vi "FPGA_I2C_Write Byte.vi"(8 "Data":u8, 9 "Wait Time/2":u32, 10 "Wait Time":u32, 11 "IO Cluster":T1) -> (2 "Done?":bool, 3 "Ack":bool)   [LabVIEW 2020]
doc: "Writes a single byte to an I2C slave device on a single port."
uses:
  Controls/FPGA_I2C IO Cluster.ctl
  Controls/FPGA I2C_Write Byte State.ctl
  <vilib>/rvi/eio/common/nirviEmuTemplateMethod_errors.vi
  <vilib>/eio/EIOMethodNode/EIOMethodNode.xnode
  <vilib>/eio/EIONode/EIONode.xnode
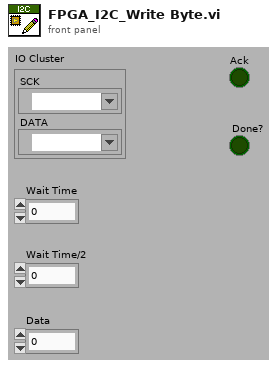
[diagram p1: front panel]
types:
  T1 = typedef "FPGA_I2C IO Cluster.ctl" = cluster{"SCK":refnum<k21>, "DATA":refnum<k21>}
  T2 = typedef "FPGA I2C_Write Byte State.ctl" = enum16{"Latch DATA", "Set DATA", "Wait Half 1", "Set SCK High 1", "Wait 1", "Set SCK Low 1", "Wait Half 2", "Release DATA", "Wait Half 3", "Set SCK High 2", "Wait Half 4", "Read Ack Bit", "Wait Half 5", "Set SCK Low 2", "Wait 2", "Stop"}
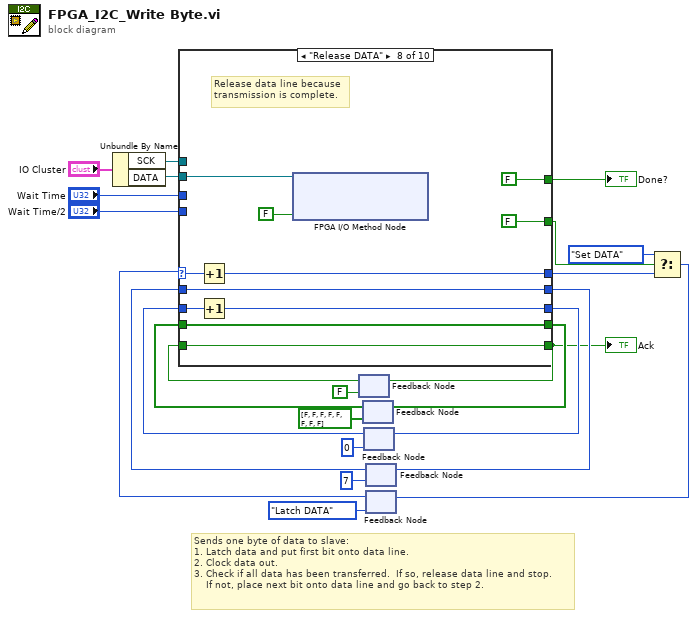
[diagram p0: block diagram]
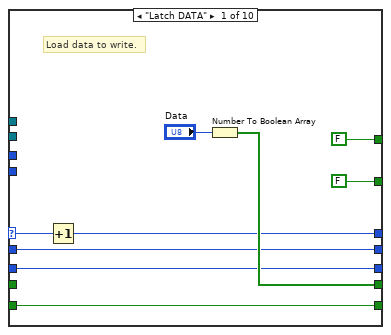
[diagram p2: hidden frame]
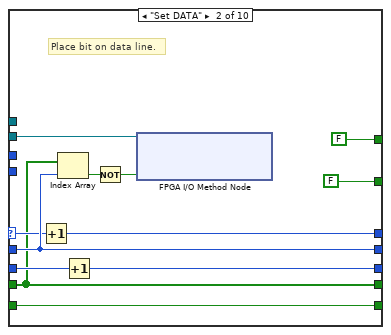
[diagram p3: hidden frame]
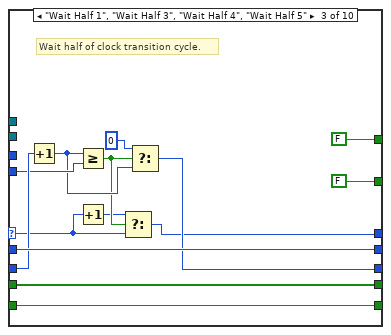
[diagram p4: hidden frame]
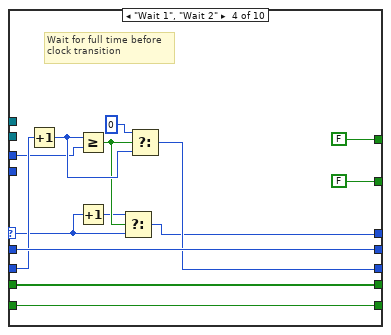
[diagram p5: hidden frame]
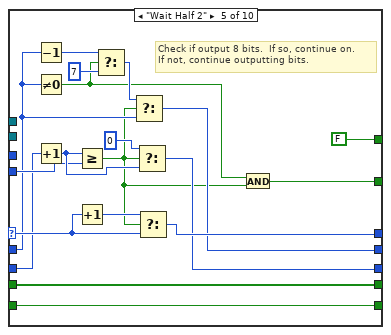
[diagram p6: hidden frame]
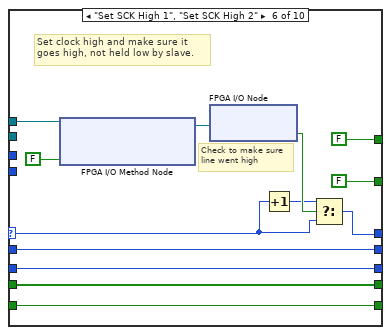
[diagram p7: hidden frame]
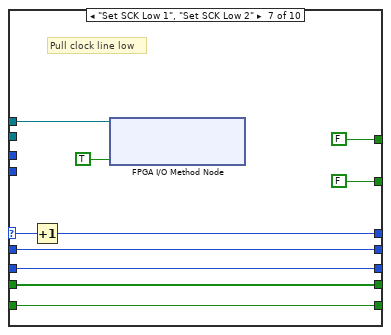
[diagram p8: hidden frame]
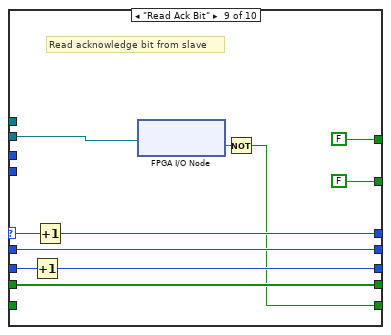
[diagram p9: hidden frame]
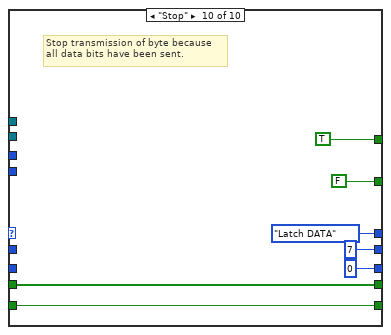
[diagram p10: hidden frame]
diagram:
  # "Sends one byte of data to slave:\n1. Latch data and put first bit onto data line.\n2. Clock data out.\n3. Check if all data has been transferred.  If so, release data line and stop.\n    If not, place next bit onto data line and go back to step 2."
  n1 = Unbundle By Name("IO Cluster") -> ("SCK"=w9:refnum<k21>, "DATA"=w10:refnum<k21>)
  n2 = feedback #1(FALSE) -> (w2:bool)
  n3 = feedback #2(bool[] [FALSE, FALSE, FALSE, FALSE, FALSE, FALSE, FALSE, FALSE] ("Boolean array")) -> (w6:bool[])
  n4 = feedback #3(u32 0) -> (w16:u32)
  n5 = feedback #4(i16 7) -> (w23:i16)
  n6 = feedback #5(FPGA_I2C_Write_Byte_State."Latch DATA" ("Enum")) -> (w4:T2)
  n7 = case shown="\"Release DATA\"" w4 {
    selector: w4 -> [w31 w42 w51 w66 w87 w103 w114 w123 w136 _]
    tunnel: w23 -> [w29 w44 w59 w73 w81 w105 w115 w126 w137 _]
    tunnel: [w29 w44 w59 w73 w80 w105 w115 w126 w137 i16 7 ("f")] -> w22
    tunnel: [FALSE FALSE FALSE FALSE w77 FALSE FALSE FALSE FALSE FALSE] -> w18
    tunnel: [FALSE FALSE FALSE FALSE FALSE FALSE FALSE FALSE FALSE TRUE] -> w20
    tunnel: [w28 w39 w54 w69 w83 w100 w111 w124 w133 u32 0 ("t")] -> w17
    tunnel: w16 -> [w28 w43 w58 w72 w84 w100 w111 w125 w134 _]
    tunnel: "Wait Time/2" -> [_ _ w57 _ w85 _ _ _ _ _]
    tunnel: [w30 w41 w50 w65 w86 w101 w113 w122 w135 FPGA_I2C_Write_Byte_State."Latch DATA" ("Enum")] -> w14
    tunnel: "Wait Time" -> [_ _ _ w64 _ _ _ _ _ _]
    tunnel: w10 -> [_ w38 _ _ _ _ _ w120 w132 _]
    tunnel: w9 -> [_ _ _ _ _ w95 w110 _ _ _]
    tunnel: [w32 w37 w49 w63 w76 w99 w109 w119 w131 w140] -> w7
    tunnel: w6 -> [_ w37 w49 w63 w76 w99 w109 w119 w131 w140]
    tunnel: w2 -> [w25 w34 w46 w60 w74 w93 w106 w116 _ w138]
    tunnel: [w25 w34 w46 w60 w74 w93 w106 w116 w127 w138] -> w1
    frame "Latch DATA" {
      # "Load data to write."
      n8 = Increment(x=w31) -> (x+1=w30:T2)
      n9 = Number To Boolean Array(number="Data") -> (Boolean array=w32:bool[])
    }
    frame "Set DATA" {
      # "Place bit on data line."
      n10 = Increment(x=w42) -> (x+1=w41:T2)
      n11 = Index Array(array=w37, index=w44) -> (element=w45:bool)
      n12 = Increment(x=w43) -> (x+1=w39:u32)
      n13 = Not(x=w45) -> (.not. x?=w40:bool)
      n14 = xnode "FPGA I/O Method Node"("FPGA I/O In"=w38, "Enable"=w40) -> ()  [unwired: 1 out]
    }
    frame "Wait Half 1", "Wait Half 3", "Wait Half 4", "Wait Half 5" {
      # "Wait half of clock transition cycle."
      n15 = Increment(x=w58) -> (x+1=w56:u32)
      n16 = Greater Or Equal?(x=w56, y=w57) -> (x >= y?=w53:bool)
      n17 = Increment(x=w51) -> (x+1=w52:T2)
      n18 = Select(t=w52, s=w53, f=w51) -> (s? t:f=w50:T2)
      n19 = Select(t=u32 0, s=w53, f=w56) -> (s? t:f=w54:u32)
    }
    frame "Wait 1", "Wait 2" {
      # "Wait for full time before\nclock transition"
      n20 = Increment(x=w72) -> (x+1=w71:u32)
      n21 = Greater Or Equal?(x=w71, y=w64) -> (x >= y?=w68:bool)
      n22 = Increment(x=w66) -> (x+1=w67:T2)
      n23 = Select(t=w67, s=w68, f=w66) -> (s? t:f=w65:T2)
      n24 = Select(t=u32 0, s=w68, f=w71) -> (s? t:f=w69:u32)
    }
    frame "Wait Half 2" {
      # "Check if output 8 bits.  If so, continue on.\nIf not, continue outputting bits."
      n25 = Decrement(x=w81) -> (x-1=w91:i16)
      n26 = Not Equal To 0?(x=w81) -> (x != 0?=w78:bool)
      n27 = Increment(x=w84) -> (x+1=w90:u32)
      n28 = Greater Or Equal?(x=w90, y=w85) -> (x >= y?=w79:bool)
      n29 = Increment(x=w87) -> (x+1=w88:T2)
      n30 = Select(t=w91, s=w78, f=i16 7) -> (s? t:f=w82:i16)
      n31 = Select(t=w82, s=w79, f=w81) -> (s? t:f=w80:i16)
      n32 = Select(t=u32 0, s=w79, f=w90) -> (s? t:f=w83:u32)
      n33 = Select(t=w88, s=w79, f=w87) -> (s? t:f=w86:T2)
      n34 = And(x=w78, y=w79) -> (x .and. y?=w77:bool)
    }
    frame "Set SCK High 1", "Set SCK High 2" {
      # "Set clock high and make sure it\ngoes high, not held low by slave."
      # "Check to make sure line went high"
      n35 = xnode "FPGA I/O Method Node"("FPGA I/O In"=w95, "Enable"=FALSE) -> ("FPGA I/O Out"=w94:refnum<k21>)
      n36 = xnode "FPGA I/O Node"("FPGA I/O In"=w94) -> ("I/O Item"=w104:bool)  [unwired: 1 out]
      n37 = Increment(x=w103) -> (x+1=w102:T2)
      n38 = Select(t=w102, s=w104, f=w103) -> (s? t:f=w101:T2)
    }
    frame "Set SCK Low 1", "Set SCK Low 2" {
      # "Pull clock line low"
      n39 = Increment(x=w114) -> (x+1=w113:T2)
      n40 = xnode "FPGA I/O Method Node"("FPGA I/O In"=w110, "Enable"=TRUE) -> ()  [unwired: 1 out]
    }
    frame "Release DATA" {
      # "Release data line because\ntransmission is complete."
      n41 = Increment(x=w123) -> (x+1=w122:T2)
      n42 = Increment(x=w125) -> (x+1=w124:u32)
      n43 = xnode "FPGA I/O Method Node"("FPGA I/O In"=w120, "Enable"=FALSE) -> ()  [unwired: 1 out]
    }
    frame "Read Ack Bit" {
      # "Read acknowledge bit from slave"
      n44 = Increment(x=w134) -> (x+1=w133:u32)
      n45 = Increment(x=w136) -> (x+1=w135:T2)
      n46 = xnode "FPGA I/O Node"("FPGA I/O In"=w132) -> ("I/O Item"=w128:bool)  [unwired: 1 out]
      n47 = Not(x=w128) -> (.not. x?=w127:bool)
    }
    frame "Stop" {
      # "Stop transmission of byte because\nall data bits have been sent."
    }
  }
  "Done?" <- w20
  "Ack" <- w1
  n48 = feedback-in #1(w1) -> ()
  n49 = feedback-in #2(w7) -> ()
  n50 = feedback-in #3(w17) -> ()
  n51 = feedback-in #4(w22) -> ()
  n52 = Select(t=FPGA_I2C_Write_Byte_State."Set DATA" ("Enum"), s=w18, f=w14) -> (s? t:f=w21:T2)
  n53 = feedback-in #5(w21) -> ()
